vi "auto_ir_bridgeBack.vi"() -> ()   [LabVIEW 2012, in "BlockParty4150.lvrbt"]
uses:
  BlockParty4150.lvrbt
  <vilib>/NXT/Subs/LVHSConnector.ctl
  <vilib>/NXT/LegoClasses/BrickReference/BrickReference.lvclass
  <vilib>/NXT/Block Support/NXT_ButtonSelector.ctl
  <vilib>/NXT/HiTechnic/HiTechnic Controls/HiTechnic Port.ctl
  <vilib>/NXT/Block Support/NXT_InputPort.ctl
  <vilib>/NXT/Hardware/Plugins/Tetrix 180 deg Servo/Tetrix180ServoAddress.ctl
  <vilib>/NXT/Hardware/Plugins/Tetrix DC Motor/TetrixDCMotorAddress.ctl
  <vilib>/NXT/Dual Mode Library/Display/drawText.vi
  <vilib>/NXT/Dual Mode Library/Sound/Tone.vi
  <vilib>/NXT/NXTIO Xnodes/NXTIONodeSubVIs/TETRIX IO Move Servos.vi
  <vilib>/NXT/Dual Mode Library/Waits/Wait_Num(msec).vi
  <vilib>/NXT/Dual Mode Library/prims/inRangeAndCoerce/inRangeAndCoerce_int.vi
  <vilib>/NXT/Dual Mode Library/Display/drawNumber.vi
  <vilib>/NXT/NXTIO Xnodes/NXTIONodeSubVIs/TETRIX IO Move DC Motors.vi
  <vilib>/NXT/NXTIO Xnodes/NXTIONodeSubVIs/TETRIX IO Stop DC Motors.vi
  <vilib>/NXT/NXTIO Xnodes/AddressXNode/NXTIOAddress.xnode
  <vilib>/NXT/NXTIO Xnodes/NXTIOXNode/NXTIO.xnode
panel:
  out "Enabled":bool
  out "iter":i32
  out "NXT":T1
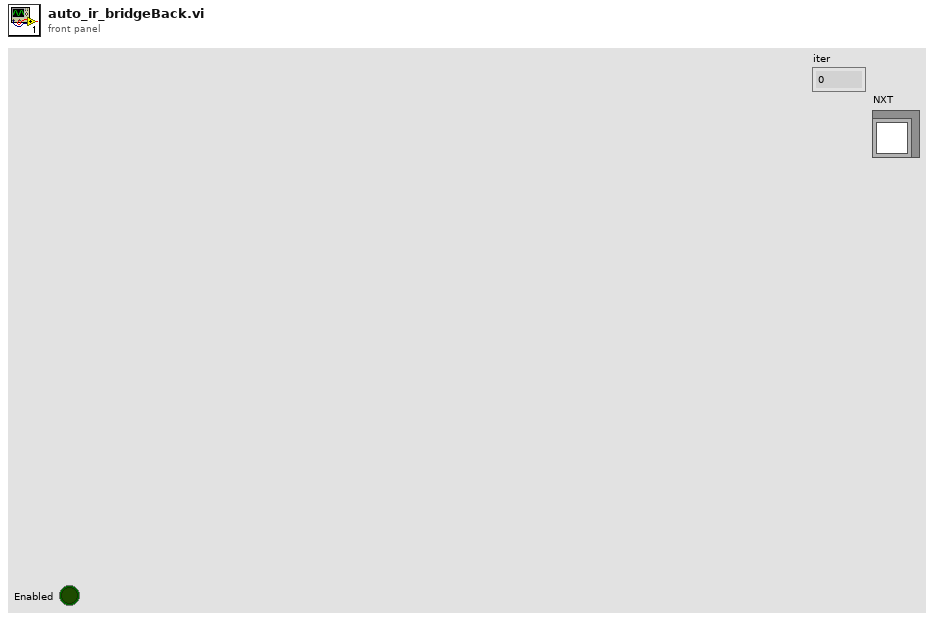
[diagram p1: front panel]
types:
  T1 = typedef "LVHSConnector.ctl" = refnum<class "BrickReference.lvclass">
  T2 = typedef "NXT_ButtonSelector.ctl" = u16
  T3 = typedef "Tetrix180ServoAddress.ctl" = i16
  T4 = typedef "TetrixDCMotorAddress.ctl" = i16
  T5 = typedef "HiTechnic Port.ctl" = cluster{"Port":T6, "MUX Port":u8}
  T6 = typedef "NXT_InputPort.ctl" = u8
  T7 = cluster{"Direction (0-9)":i16, "Signal Strength (Array)":u8[]}
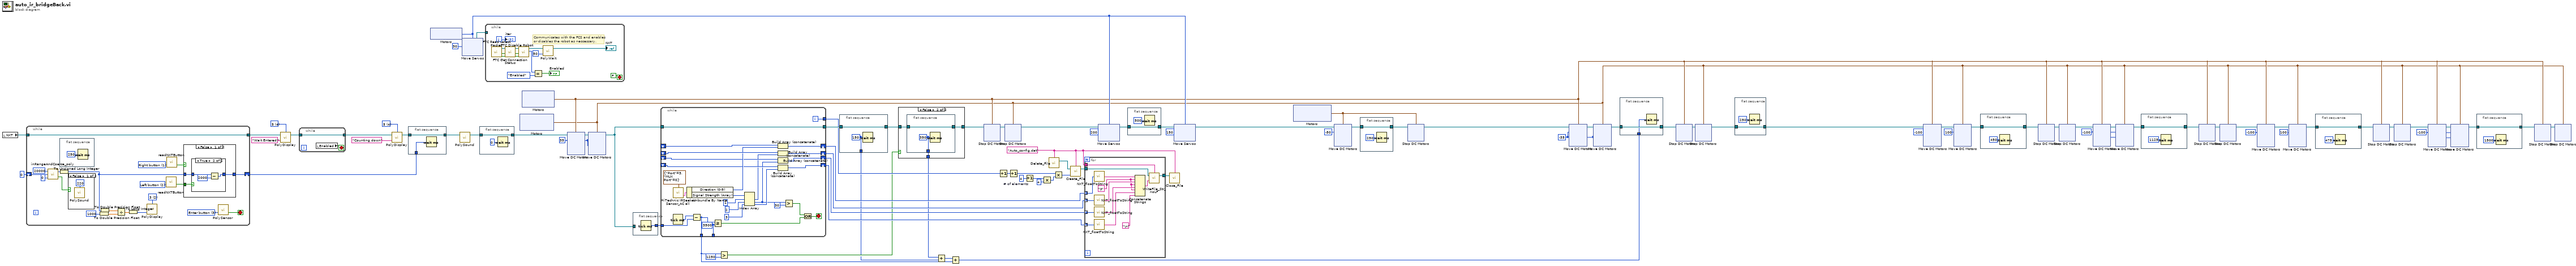
[diagram p0: block diagram]
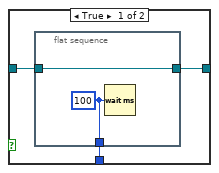
[diagram p2: hidden frame]
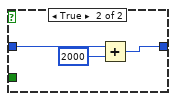
[diagram p5: hidden frame]
diagram:
  w7 = i8 -50 ("Power/Speed 1")
  w12 = i8 -35 ("Power/Speed 1")
  w28 = i8 -100 ("Power/Speed 1")
  w34 = i8 100 ("Power/Speed 1")
  w33 = i8 -100 ("Power/Speed 1")
  w40 = i8 -100 ("Power/Speed 1")
  w46 = i8 100 ("Power/Speed 1")
  w45 = i8 -100 ("Power/Speed 1")
  w63 = 4  # # of elements
  w60 = "Auto_config.dat" ("Filename")
  w76 = i8 35 ("Power/Speed 1")
  w84 = i16 4 items=["1", "2", "3", "4", "5", "6", "7", "8"] ("Line")
  w85 = i16 4 items=["1", "2", "3", "4", "5", "6", "7", "8"] ("Line")
  n1 = local read "NXT"() -> (w78:T1)
  n2 = while {
    tunnel: [w113] -> w87
    tunnel: w78 -> [w113]
    shift-right: [w106] -> w88
    shift-left: u32 0 ("Power/Speed 1") -> [w99]
    stop <- w111 stop-if-true
    w105 = i16 2 items=["1", "2", "3", "4", "5", "6", "7", "8"] ("Line")
    w108 = T2 1 items=["Enter button"=3, "Left button"=2, "Right button"=1] ("Button (Enter button)")
    w107 = T2 2 items=["Enter button"=3, "Left button"=2, "Right button"=1] ("Button (Enter button)")
    w112 = T2 3 items=["Enter button"=3, "Left button"=2, "Right button"=1] ("Button (Enter button)")
    n3 = call-poly <vilib>:"inRangeAndCoerce_poly.vi"("lower limit"=0, "x"=w99, "upper limit"=20000) -> ("In Range?"=w94:bool, "coerced(x)"=w96:i32)
    n4 = To Unsigned Long Integer(number=w96) -> (unsigned 32bit integer=w95:u32)
    n5 = flat-sequence {
      frame #0 {
        n6 = Wait (ms)(milliseconds to wait=u32 250) -> ()  [unwired: 1 out]
      }
    }
    n7 = case shown="False" w94 {
      frame False {
        n8 = call-poly <vilib>:"PolySound.vi"("Tone (440 Hz)"=u16 220) -> ()  [unwired: 3 in, 1 out]
      }
      frame True {
      }
    }
    n9 = To Double Precision Float(number=u32 1000 ("Power/Speed 1")) -> (double precision float=w100:dbl)
    n10 = To Double Precision Float(number=w95) -> (double precision float=w102:dbl)
    n11 = Divide(x=w102, y=w100) -> (x/y=w103:dbl)
    n12 = To Long Integer(number=w103) -> (32bit integer=w101:i32)
    n13 = call-poly <vilib>:"PolyDisplay.vi"("number"=w101, "Line"=w105) -> ()  [unwired: 2 in, 1 out]
    n14 = call <vilib>:"readNXTButton.vi"("Button (Enter button)"=w107) -> ("Yes/No"=w110:bool)  [unwired: 2 in, 1 out]
    n15 = call <vilib>:"readNXTButton.vi"("Button (Enter button)"=w108) -> ("Yes/No"=w109:bool)  [unwired: 2 in, 1 out]
    n16 = case shown="False" w109 {
      tunnel: w110 -> [w118 _]
      tunnel: [w117 w124] -> w106
      tunnel: w95 -> [w116 w125]
      frame False {
        n17 = case shown="True" w118 {
          tunnel: [w119 w121] -> w117
          tunnel: w116 -> [w119 w122]
          frame False {
          }
          frame True {
            n18 = Subtract(x=w122, y=u32 2000) -> (x-y=w121:u32)
          }
        }
      }
      frame True {
        n19 = Add(x=w125, y=u32 2000) -> (x+y=w124:u32)
      }
    }
    n20 = call-poly <vilib>:"PolySensor.vi"("Button (Enter button)"=w112) -> ("Yes/No"=w111:bool)  [unwired: 2 in, 1 out]
  }
  n21 = call-poly <vilib>:"PolyDisplay.vi"("Text"="Wait Entered!", "NXT"=w87, "Line"=w85) -> ("NXT"=w80:T1)  [unwired: 1 in]
  n22 = while {
    tunnel: [w126] -> w79
    tunnel: w80 -> [w126]
    stop <- w127 stop-if-true
    n23 = local read "Enabled"() -> (w127:bool)
  }
  n24 = call-poly <vilib>:"PolyDisplay.vi"("Text"="Counting down", "NXT"=w79, "Line"=w84) -> ("NXT"=w82:T1)  [unwired: 1 in]
  n25 = flat-sequence {
    tunnel: w82 -> [w129]
    tunnel: [w129] -> w90
    tunnel: w88 -> [w128]
    frame #0 {
      n26 = Wait (ms)(milliseconds to wait=w128) -> ()  [unwired: 1 out]
    }
  }
  n27 = xnode "Motors"() -> ("Motor"=w91:T3)
  n28 = call-poly <vilib>:"PolySound.vi"("NXT"=w90) -> ("NXT"=w81:T1)  [unwired: 3 in]
  n29 = xnode "Move Servos"("Position 1"=u8 30, "Servos"=w91) -> ("NXT"=w92:T1)  [unwired: 1 in]
  n30 = flat-sequence {
    tunnel: w81 -> [w131]
    tunnel: [w131] -> w73
    frame #0 {
      n31 = Wait (ms)(milliseconds to wait=u32 0) -> ()  [unwired: 1 out]
    }
  }
  n32 = while {
    tunnel: w92 -> [_]
    i -> [w133]
    stop <- FALSE stop-if-true
    # "Communicates with the FCS and enables \nor disables the robot as neccessary."
    n33 = call <vilib>:"FTC Read Latest Packet.vi"() -> ("Packet Received?"=w143:bool, "Stopped?"=w142:bool, "NXT"=w145:T1)  [unwired: 6 in, 3 out]
    n34 = call <vilib>:"FTC Get Connection Status.vi"("Packet Received?"=w143, "Stopped?"=w142, "NXT"=w145) -> ("Online?"=w135:bool, "Stopped?"=w136:bool, "NXT"=w144:T1)  [unwired: 5 in]
    n35 = call <vilib>:"FTC Disable Robot.vi"("Online?"=w135, "Stopped?"=w136, "NXT"=w144) -> ("Enabled?"=w139:enum16{"Disabled", "Enabled"}, "NXT"=w141:T1)  [unwired: 3 in]
    n36 = Equal?(x=w139, y=enum16{"Disabled", "Enabled"}."Enabled") -> (x = y?=→"Enabled":bool)
    n37 = call-poly <vilib>:"PolyWait.vi"("Time (100 msec)"=u32 50 ("Time (msec)"), "NXT"=w141) -> ("NXT"=→"NXT":T1)  [unwired: 2 in]
    "iter" <- w133
  }
  n38 = xnode "Motors"() -> ("Motor"=w69:cluster{"TetrixDCMotor":T4, "TetrixDCMotor":T4})
  n39 = xnode "Motors"() -> ("Motor"=w70:cluster{"TetrixDCMotor":T4, "TetrixDCMotor":T4})
  n40 = xnode "Move DC Motors"("Power/Speed 2"=w76, "Power/Speed 1"=w76, "Motors"=w70, "NXT"=w73) -> ("NXT"=w77:T1)
  n41 = xnode "Move DC Motors"("Power/Speed 2"=w76, "Power/Speed 1"=w76, "Motors"=w69, "NXT"=w77) -> ("NXT"=w74:T1)
  n42 = flat-sequence {
    tunnel: [w146] -> w72
    tunnel: w74 -> [_]
    frame #0 {
      n43 = Tick Count (ms)() -> (millisecond timer value=w146:u32)
    }
  }
  n44 = while {
    tunnel: [w173] -> w21
    shift-right: [w172] -> w57
    shift-left: _ -> [w171]
    shift-right: [w169] -> w56
    shift-left: _ -> [w170]
    shift-right: [w158] -> w55
    shift-left: _ -> [w161]
    shift-right: [w157] -> w54
    shift-left: _ -> [w160]
    tunnel: w74 -> [w156]
    tunnel: [w156] -> w71
    tunnel: w72 -> [w149]
    tunnel: [w148] -> w10
    tunnel: [w147] -> _
    i -> [w173]
    stop <- w153 stop-if-true
    w147 = u32 3500 ("y")
    n45 = Tick Count (ms)() -> (millisecond timer value=w174:u32)
    n46 = call <vilib>:"HiTechnic IRSeeker Sensor_AC all.vi"("Port/MUX"=T5 {"Port"=3, "MUX Port"=0}) -> ("All Info"=w168:T7)  [unwired: 2 in, 1 out]
    n47 = Unbundle By Name(w168) -> ("Direction (0-9)"=w164:i16, "Signal Strength (Array)"=w167:u8[])
    n48 = Subtract(x=w174, y=w149) -> (x-y=w148:u32)
    n49 = Greater Or Equal?(x=w148, y=w147) -> (x >= y?=w151:bool)
    n50 = Index Array(array=w167, index #1=1 ("index"), index #2=2 ("index"), index #3=3 ("index")) -> (element #1=w155:u8, element #2=w150:u8, element #3=w159:u8)
    n51 = Build Array (concatenate)(w171, w164) -> (w172:i16[])
    n52 = Build Array (concatenate)(w170, w155) -> (w169:u8[])
    n53 = Build Array (concatenate)(w161, w150) -> (w158:u8[])
    n54 = Build Array (concatenate)(w160, w159) -> (w157:u8[])
    n55 = Greater?(x=w150, y=u8 30) -> (0:w152:bool)
    n56 = Or(x=w152, y=w151) -> (x .or. y?=w153:bool)
  }
  n57 = Greater?(x=w10, y=u32 1250) -> (0:w17:bool)
  n58 = flat-sequence {
    tunnel: [w176] -> w20
    tunnel: w71 -> [w176]
    tunnel: [w175] -> w15
    frame #0 {
      w175 = u32 150 ("milliseconds to wait")
      n59 = Wait (ms)(milliseconds to wait=w175) -> ()  [unwired: 1 out]
    }
  }
  n60 = case shown="False" w17 {
    tunnel: w20 -> [w179 w184]
    tunnel: [w178 w183] -> w19
    tunnel: [w177 w182] -> w16
    frame True {
      n61 = flat-sequence {
        tunnel: [w181] -> w177
        tunnel: [w180] -> w178
        tunnel: w179 -> [w180]
        frame #0 {
          w181 = u32 100 ("milliseconds to wait")
          n62 = Wait (ms)(milliseconds to wait=w181) -> ()  [unwired: 1 out]
        }
      }
    }
    frame False {
      n63 = flat-sequence {
        tunnel: [w186] -> w182
        tunnel: [w185] -> w183
        tunnel: w184 -> [w185]
        frame #0 {
          w186 = u32 350 ("milliseconds to wait")
          n64 = Wait (ms)(milliseconds to wait=w186) -> ()  [unwired: 1 out]
        }
      }
    }
  }
  n65 = Add(x=w16, y=w15) -> (x+y=w11:u32)
  n66 = Add(x=w11, y=w10) -> (x+y=w9:u32)
  n67 = xnode "Stop DC Motors"("Motors"=w70, "NXT"=w19) -> ("NXT"=w75:T1)
  n68 = Increment(x=w21) -> (x+1=w61:i32)
  n69 = xnode "Stop DC Motors"("Motors"=w69, "NXT"=w75) -> ("NXT"=w49:T1)
  n70 = Increment(x=w61) -> (x+1=w67:i32)
  n71 = Increment(x=w63) -> (x+1=w64:i32)
  n72 = Multiply(x=w64, y=u32 4) -> (x*y=w65:u32)
  n73 = call <vilib>:"Delete_File.vi"("Filename"=w60) -> ("NXT"=w68:T1)  [unwired: 3 in]
  n74 = Multiply(x=w67, y=w65) -> (x*y=w58:u32)
  n75 = call <vilib>:"Create_File.vi"("File Size (256)"=w58, "NXT"=w68, "Filename"=w60) -> ("NXT"=w59:T1)  [unwired: 1 out]
  n76 = for {
    tunnel: w60 -> [w200]
    tunnel: w59 -> [w199]
    tunnel: [w198] -> w62
    tunnel: w57 -> [w197] mode=indexing
    tunnel: w56 -> [w195] mode=indexing
    tunnel: w55 -> [w188] mode=indexing
    tunnel: w54 -> [w187] mode=indexing
    w191 = "\t" ("string")
    n77 = call <vilib>:"NXT_floatToString.vi"("number"=w197) -> ("string"=w194:string)
    n78 = call <vilib>:"NXT_floatToString.vi"("number"=w195) -> ("string"=w193:string)
    n79 = call <vilib>:"NXT_floatToString.vi"("number"=w188) -> ("string"=w192:string)
    n80 = call <vilib>:"NXT_floatToString.vi"("number"=w187) -> ("string"=w190:string)
    n81 = Concatenate Strings(w194, w191, w193, w191, w192, w191, w190, "\n") -> (w196:string)
    n82 = call <vilib>:"WriteFile_Str_noLF.vi"("String"=w196, "NXT"=w199, "Filename"=w200) -> ("NXT"=w198:T1)  [unwired: 1 in]
  }
  n83 = xnode "Move Servos"("Position 1"=u8 200, "Servos"=w91, "NXT"=w49) -> ("NXT"=w52:T1)
  n84 = flat-sequence {
    tunnel: [w201] -> w50
    tunnel: w52 -> [w201]
    frame #0 {
      n85 = Wait (ms)(milliseconds to wait=u32 500) -> ()  [unwired: 1 out]
    }
  }
  n86 = call <vilib>:"Close_File.vi"("NXT"=w62, "Filename"=w60) -> ()  [unwired: 2 in, 1 out]
  n87 = xnode "Move Servos"("Position 1"=u8 150, "Servos"=w91, "NXT"=w50) -> ("NXT"=w2:T1)
  n88 = xnode "Motors"() -> ("Motor"=w4:cluster{"TetrixDCMotor":T4, "TetrixDCMotor":T4})
  n89 = xnode "Move DC Motors"("Power/Speed 2"=w7, "Power/Speed 1"=w7, "Motors"=w4, "NXT"=w2) -> ("NXT"=w6:T1)
  n90 = flat-sequence {
    tunnel: w6 -> [w203]
    tunnel: [w203] -> w5
    frame #0 {
      n91 = Wait (ms)(milliseconds to wait=u32 250) -> ()  [unwired: 1 out]
    }
  }
  n92 = xnode "Stop DC Motors"("Motors"=w4, "NXT"=w5) -> ("NXT"=w3:T1)
  n93 = xnode "Move DC Motors"("Power/Speed 2"=w12, "Power/Speed 1"=w12, "Motors"=w70, "NXT"=w3) -> ("NXT"=w14:T1)
  n94 = xnode "Move DC Motors"("Power/Speed 2"=w12, "Power/Speed 1"=w12, "Motors"=w69, "NXT"=w14) -> ("NXT"=w13:T1)
  n95 = flat-sequence {
    tunnel: [w206] -> w47
    tunnel: w13 -> [w206]
    tunnel: w9 -> [w205]
    frame #0 {
      n96 = Wait (ms)(milliseconds to wait=w205) -> ()  [unwired: 1 out]
    }
  }
  n97 = xnode "Stop DC Motors"("Motors"=w70, "NXT"=w47) -> ("NXT"=w48:T1)
  n98 = xnode "Stop DC Motors"("Motors"=w69, "NXT"=w48) -> ("NXT"=w8:T1)
  n99 = flat-sequence {
    tunnel: [w208] -> w1
    tunnel: w8 -> [w208]
    frame #0 {
      n100 = Wait (ms)(milliseconds to wait=u32 250) -> ()  [unwired: 1 out]
    }
  }
  n101 = xnode "Move DC Motors"("Power/Speed 2"=w45, "Power/Speed 1"=w45, "Motors"=w70, "NXT"=w1) -> ("NXT"=w44:T1)
  n102 = xnode "Move DC Motors"("Power/Speed 2"=w46, "Power/Speed 1"=w46, "Motors"=w69, "NXT"=w44) -> ("NXT"=w41:T1)
  n103 = flat-sequence {
    tunnel: [w209] -> w43
    tunnel: w41 -> [w209]
    frame #0 {
      n104 = Wait (ms)(milliseconds to wait=u32 450) -> ()  [unwired: 1 out]
    }
  }
  n105 = xnode "Stop DC Motors"("Motors"=w70, "NXT"=w43) -> ("NXT"=w42:T1)
  n106 = xnode "Stop DC Motors"("Motors"=w69, "NXT"=w42) -> ("NXT"=w35:T1)
  n107 = xnode "Move DC Motors"("Power/Speed 2"=w40, "Power/Speed 1"=w40, "Motors"=w70, "NXT"=w35) -> ("NXT"=w39:T1)
  n108 = xnode "Move DC Motors"("Power/Speed 2"=w40, "Power/Speed 1"=w40, "Motors"=w69, "NXT"=w39) -> ("NXT"=w36:T1)
  n109 = flat-sequence {
    tunnel: [w211] -> w38
    tunnel: w36 -> [w211]
    frame #0 {
      n110 = Wait (ms)(milliseconds to wait=u32 1125) -> ()  [unwired: 1 out]
    }
  }
  n111 = xnode "Stop DC Motors"("Motors"=w70, "NXT"=w38) -> ("NXT"=w37:T1)
  n112 = xnode "Stop DC Motors"("Motors"=w69, "NXT"=w37) -> ("NXT"=w22:T1)
  n113 = xnode "Move DC Motors"("Power/Speed 2"=w33, "Power/Speed 1"=w33, "Motors"=w70, "NXT"=w22) -> ("NXT"=w32:T1)
  n114 = xnode "Move DC Motors"("Power/Speed 2"=w34, "Power/Speed 1"=w34, "Motors"=w69, "NXT"=w32) -> ("NXT"=w29:T1)
  n115 = flat-sequence {
    tunnel: [w213] -> w31
    tunnel: w29 -> [w213]
    frame #0 {
      n116 = Wait (ms)(milliseconds to wait=u32 475) -> ()  [unwired: 1 out]
    }
  }
  n117 = xnode "Stop DC Motors"("Motors"=w70, "NXT"=w31) -> ("NXT"=w30:T1)
  n118 = xnode "Stop DC Motors"("Motors"=w69, "NXT"=w30) -> ("NXT"=w23:T1)
  n119 = xnode "Move DC Motors"("Power/Speed 2"=w28, "Power/Speed 1"=w28, "Motors"=w70, "NXT"=w23) -> ("NXT"=w27:T1)
  n120 = xnode "Move DC Motors"("Power/Speed 2"=w28, "Power/Speed 1"=w28, "Motors"=w69, "NXT"=w27) -> ("NXT"=w24:T1)
  n121 = flat-sequence {
    tunnel: [w215] -> w26
    tunnel: w24 -> [w215]
    frame #0 {
      n122 = Wait (ms)(milliseconds to wait=u32 1500) -> ()  [unwired: 1 out]
    }
  }
  n123 = xnode "Stop DC Motors"("Motors"=w70, "NXT"=w26) -> ("NXT"=w25:T1)
  n124 = xnode "Stop DC Motors"("Motors"=w69, "NXT"=w25) -> ()  [unwired: 1 out]
